vi "PID_Calculation.vi"(4 "Ki":dbl=0.01, 5 "Kp":dbl=30.0, 6 "Kd":dbl=0.03, 7 "Angle":ext, 9 "sum_[e(t)*dt]":ext, 10 "e(t-1)":ext, 11 "milliseconds to wait in":ext) -> (0 "PID":ext, 1 "sum_[e(t)*dt] + new_[e(t)*dt]":ext, 2 "PID":dbl=47.931426005026836, 3 "e(t)":ext)   [LabVIEW 2021]
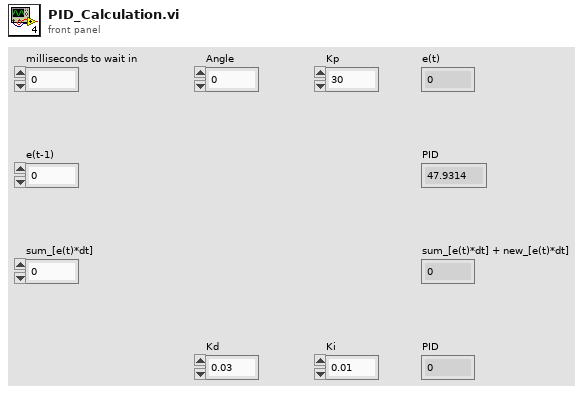
[diagram p1: front panel]
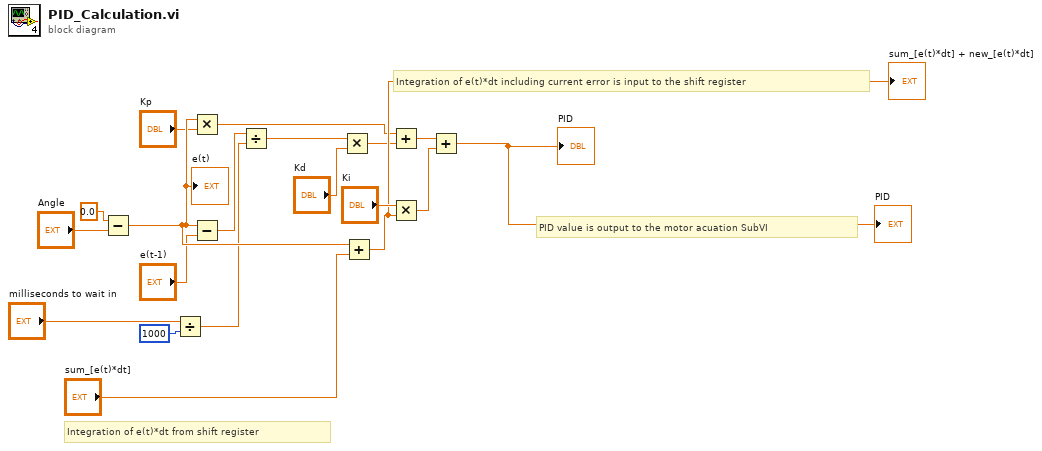
[diagram p0: block diagram]
diagram:
  # "PID value is output to the motor acuation SubVI"
  # "Integration of e(t)*dt including current error is input to the shift register"
  # "Integration of e(t)*dt from shift register"
  n1 = Subtract(x=0.0, y="Angle") -> (x-y=w14:ext)
  "e(t)" <- w14
  n2 = Divide(x="milliseconds to wait in", y=u32 1000) -> (x/y=w11:ext)
  n3 = Multiply(x=w14, y="Kp") -> (x*y=w2:ext)
  n4 = Subtract(x=w14, y="e(t-1)") -> (x-y=w5:ext)
  n5 = Divide(x=w5, y=w11) -> (x/y=w6:ext)
  n6 = Multiply(x=w6, y="Kd") -> (x*y=w1:ext)
  n7 = Add(x=w14, y="sum_[e(t)*dt]") -> (x+y=w15:ext)
  "sum_[e(t)*dt] + new_[e(t)*dt]" <- w15
  n8 = Add(x=w2, y=w1) -> (x+y=w17:ext)
  n9 = Multiply(x="Ki", y=w15) -> (x*y=w18:ext)
  n10 = Add(x=w17, y=w18) -> (x+y=→"PID" →"PID":ext)
